vi "Stop Cooker.vi"(8 "error in (no error)":errorcluster, 11 "Direct Cooker in":refnum<class "Direct Cooker.lvclass">) -> (0 "error out":errorcluster, 2 "Finished?":bool, 3 "Direct Cooker out":refnum<class "Direct Cooker.lvclass">)   [LabVIEW 2024, in "Cooker Actor.lvlib" / "Direct Cooker.lvclass"]
uses:
  Direct Cooker.lvclass
  Direct Cooker.lvclass/Direct Cooker.ctl
  Cooker Actor/Cooker Actor.lvclass
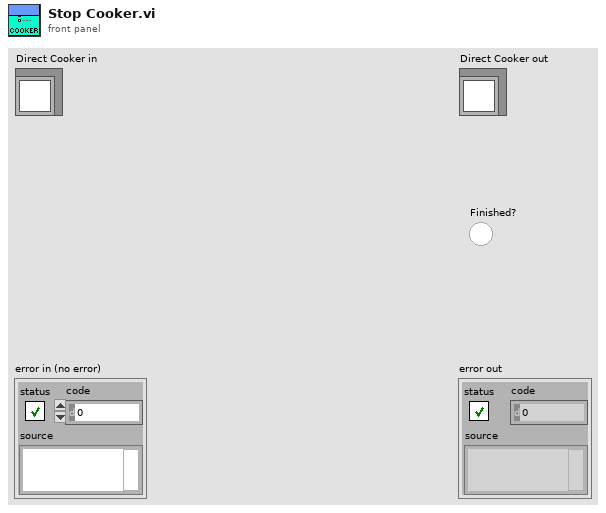
[diagram p1: front panel]
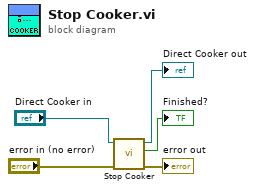
[diagram p0: block diagram]
diagram:
  n1 = call-parent "Stop Cooker.vi"("error in (no error)"="error in (no error)", "Cooker Actor in"="Direct Cooker in") -> ("error out"=→"error out":errorcluster, "Finished?"=→"Finished?":bool, "Cooker Actor out"=→"Direct Cooker out":refnum<class "Direct Cooker.lvclass">)  [unwired: 7 in]
